vi "RPC Server Template.vi"   [LabVIEW 2015, in "JSONRPC Server.lvclass"]
doc: "Use this as a starting point for the RPC Server processing loop in your application"
uses:
  JSONRPC Server.lvclass
  Request/Request.lvclass/Request.ctl
  Request/Read method.vi
  Request/Read params.vi
  Add Response (Result from Request).vi
  Add Response (Invalid Params from Request).vi
  Add Response (Server Error from Request).vi
  <vilib>/NI/JSON Support for LabVIEW/JSON Data Classes/JSON Datatype/JSON Null.lvclass
  params/params.lvclass
  Request/Request.lvclass
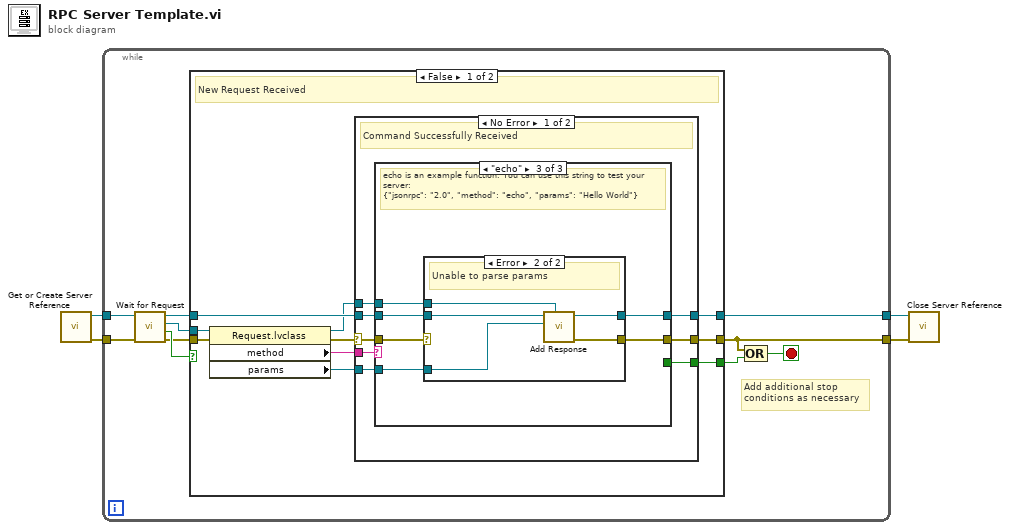
[diagram p0: block diagram]
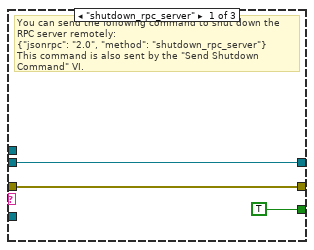
[diagram p2: hidden frame]
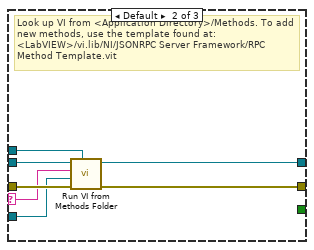
[diagram p3: hidden frame]
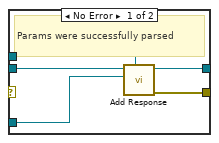
[diagram p4: hidden frame]
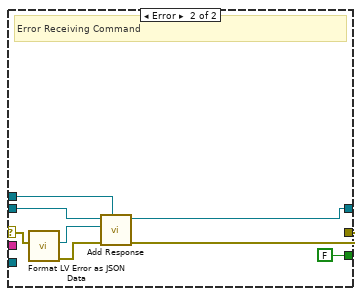
[diagram p5: hidden frame]
diagram:
  n1 = call "Get or Create Server Reference.vi"() -> ("error out"=w3:errorcluster, "Server Out"=w4:refnum<class "JSONRPC Server.lvclass">)  [unwired: 10 in]
  n2 = while {
    tunnel: w4 -> [w14]
    tunnel: w3 -> [w10]
    tunnel: [w6] -> w1
    tunnel: [w8] -> w2
    stop <- w5 stop-if-true
    # "Add additional stop\nconditions as necessary"
    n3 = call "Wait for Request.vi"("error in (no error)"=w10, "Server in"=w14) -> ("error out"=w9:errorcluster, "timed out?"=w11:bool, "Request"=w12:refnum<class "Request.lvclass">, "Server out"=w13:refnum<class "JSONRPC Server.lvclass">)  [unwired: 6 in]
    n4 = case shown="False" w11 {
      tunnel: w13 -> [w17 w67]
      tunnel: w12 -> [w24 _]
      tunnel: w9 -> [w21 w68]
      tunnel: [w19 w68] -> w6
      tunnel: [w18 _] -> w7
      tunnel: [w16 w67] -> w8
      frame False {
        # "New Request Received"
        n5 = property class="Request.lvclass"(reference=w24, error in=w21) -> (reference out=w15:refnum<class "Request.lvclass">, error out=w20:errorcluster, "method"=w23:string, "params"=w22:refnum<class "JSON Null.lvclass">)
        n6 = case shown="No Error" w20 {
          selector: w20 -> [w30 w60]
          tunnel: w23 -> [w32 _]
          tunnel: w22 -> [w31 _]
          tunnel: [w29 w63] -> w19
          tunnel: [w28 FALSE] -> w18
          tunnel: w17 -> [w27 w65]
          tunnel: [w26 w64] -> w16
          tunnel: w15 -> [w25 w66]
          frame No Error {
            # "Command Successfully Received"
            n7 = case shown="\"echo\"" w32 {
              selector: w32 -> [_ w36 _]
              tunnel: w31 -> [_ w40 w44]
              tunnel: w30 -> [w34 w42 w43]
              tunnel: [w34 w39 w46] -> w29
              tunnel: [TRUE _ _] -> w28
              tunnel: w27 -> [w33 w41 w48]
              tunnel: [w33 w38 w47] -> w26
              tunnel: w25 -> [_ w37 w45]
              frame "shutdown_rpc_server" {
                # "You can send the following command to shut down the RPC server remotely:\n{\"jsonrpc\": \"2.0\", \"method\": \"shutdown_rpc_server\"}\nThis command is also sent by the \"Send Shutdown Command\" VI."
              }
              frame Default {
                # "Look up VI from <Application Directory>/Methods. To add new methods, use the template found at:\n<LabVIEW>/vi.lib/NI/JSONRPC Server Framework/RPC Method Template.vit"
                n8 = call "Run VI from Methods Folder.vi"("Request"=w37, "error in (no error)"=w42, "params"=w40, "String"=w36, "JSONRPC Server in"=w41) -> ("error out"=w39:errorcluster, "JSONRPC Server out"=w38:refnum<class "JSONRPC Server.lvclass">)  [unwired: 5 in]
              }
              frame "echo" {
                # "echo is an example function. You can use this string to test your server:\n{\"jsonrpc\": \"2.0\", \"method\": \"echo\", \"params\": \"Hello World\"}"
                n9 = case shown="Error" w43 {
                  tunnel: w48 -> [w53 w58]
                  tunnel: [w52 w57] -> w47
                  tunnel: w44 -> [w51 w56]
                  tunnel: [w50 w55] -> w46
                  tunnel: w45 -> [w49 w54]
                  frame No Error {
                    # "Params were successfully parsed"
                    n10 = call-poly "Add Response.vi"("Request"=w49, "JSON in"=w51, "Server in"=w53) -> ("error out"=w50:errorcluster, "Server out"=w52:refnum<class "JSONRPC Server.lvclass">)  [unwired: 6 in, 1 out]
                  }
                  frame Error {
                    # "Unable to parse params"
                    n11 = call-poly "Add Response.vi"("Request"=w54, "data"=w56, "Server in"=w58) -> ("error out"=w55:errorcluster, "Server out"=w57:refnum<class "JSONRPC Server.lvclass">)  [unwired: 6 in, 1 out]
                  }
                }
              }
            }
          }
          frame Error {
            # "Error Receiving Command"
            n12 = call "Format LV Error as JSON Data.vi"("error in"=w60) -> ("error out"=w61:errorcluster, "Error Object Out"=w59:refnum<class "JSON Object.lvclass">)  [unwired: 9 in]
            n13 = call-poly "Add Response.vi"("Request"=w66, "error in (no error)"=w61, "data"=w59, "Server in"=w65) -> ("error out"=w63:errorcluster, "Server out"=w64:refnum<class "JSONRPC Server.lvclass">)  [unwired: 5 in, 1 out]
          }
        }
      }
      frame True {
        # "Timeout while waiting for new Requests"
      }
    }
    n14 = Compound Arithmetic op=OR(w6, w7) -> (w5:bool)
  }
  n15 = call-dynamic "Close Server Reference.vi"("error in (no error)"=w1, "Server in"=w2) -> ()  [unwired: 9 in, 1 out]
